vi "average_centroid.vi"(6 "input valid":bool, 9 "Average":u16, 10 "Input value":fxp<+,32,16>) -> (2 "av_ready":bool, 3 "cent_av":fxp<+,32,16>)   [LabVIEW 2020]
uses:
  <vilib>/rvi/FXPMathLib/FxpDiv/subVIs/nifxpmath_Div_SimConfig.ctl
  <vilib>/rvi/FXPMathLib/FxpDiv/simVIs/DllFxpDivTemp_sub.vi
  <vilib>/rvi/FXPMathLib/FxpAdd/XNode/nifxpmath_Add.xnode
  <vilib>/rvi/FXPMathLib/FxpDiv/XNode/nifxpmath_Div.xnode
  <vilib>/rvi/FXPMathLib/sim/FxpSim.dll
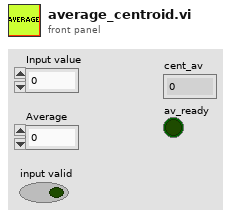
[diagram p1: front panel]
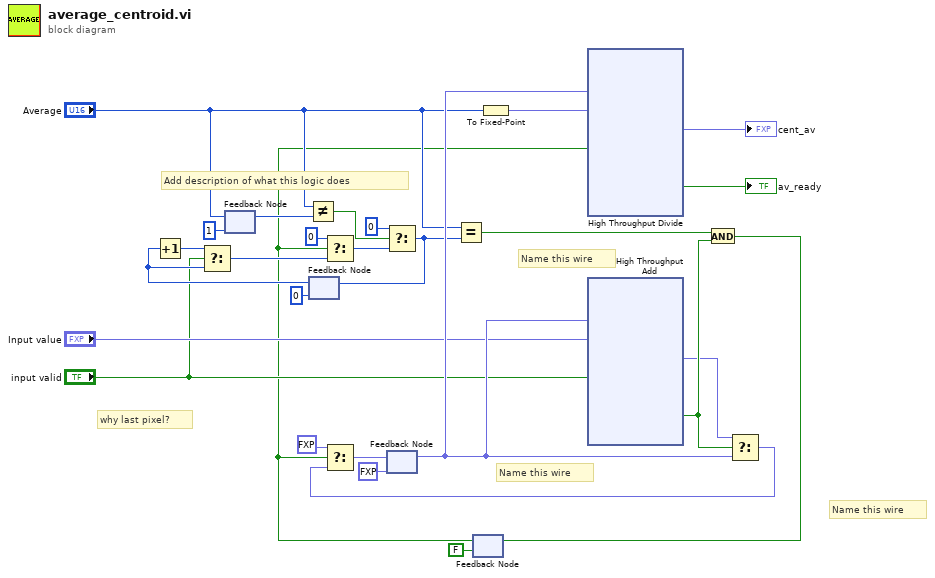
[diagram p0: block diagram]
diagram:
  # "why last pixel?"
  # "Name this wire"
  # "Name this wire"
  # "Name this wire"
  # "Add description of what this logic does"
  n1 = feedback-in #1("Average") -> ()
  n2 = feedback #1(u16 1 ("Average")) -> (w7:u16)
  n3 = Not Equal?(x="Average", y=w7) -> (x != y?=w6:bool)
  n4 = feedback #2(u16 0 ("t")) -> (w18:u16)
  n5 = Increment(x=w18) -> (x+1=w11:u16)
  n6 = Select(t=w11, s="input valid", f=w18) -> (s? t:f=w10:u16)
  n7 = feedback #3(fxp<+,32,16> 0.0 ("x+y")) -> (w26:fxp<+,32,16>)
  n8 = feedback #4(FALSE ("dv in")) -> (w2:bool)
  n9 = Select(t=u16 0, s=w2, f=w10) -> (s? t:f=w4:u16)
  n10 = Select(t=u16 0, s=w6, f=w4) -> (s? t:f=w3:u16)
  n11 = feedback-in #2(w3) -> ()
  n12 = Equal?(x="Average", y=w3) -> (x = y?=w21:bool)
  n13 = To Fixed-Point(number="Average") -> (fixed-point=w27:fxp<+,16,16>)  [unwired: 1 in]
  n14 = xnode ("High Throughput Divide")("x"=w26, "y"=w27, "input valid"=w2) -> ("x/y"=→"cent_av":fxp<+,32,16>, "output valid"=→"av_ready":bool)  [unwired: 1 in, 1 out]
  n15 = xnode ("High Throughput Add")("x"=w26, "y"="Input value", "input valid"="input valid") -> ("x+y"=w19:fxp<+,32,16>, "output valid"=w20:bool)  [unwired: 1 in, 1 out]
  n16 = And(x=w21, y=w20) -> (x .and. y?=w1:bool)
  n17 = feedback-in #4(w1) -> ()
  n18 = Select(t=w19, s=w20, f=w26) -> (s? t:f=w16:fxp<+,32,16>)
  n19 = Select(t=fxp<+,32,16> 0.0, s=w2, f=w16) -> (s? t:f=w15:fxp<+,32,16>)
  n20 = feedback-in #3(w15) -> ()
